vi "sub vi test.vi"() -> ()   [LabVIEW 2019]
uses:
  <userlib>/defectsWrapper/defectsWrapper.lvlib
panel:
  out "Image":T1(plugin-control)
  in  "margin":dbl[][](array[numeric])=[[650.0, 1550.0]]
  in  "thr":dbl[][](array[numeric])=[[900.0, 900.0, 1000.0, 1100.0, 1800.0, 1800.0, 2000.0, 2200.0]]
  in  "File Path":path
  in  "error in (no error)":errorcluster
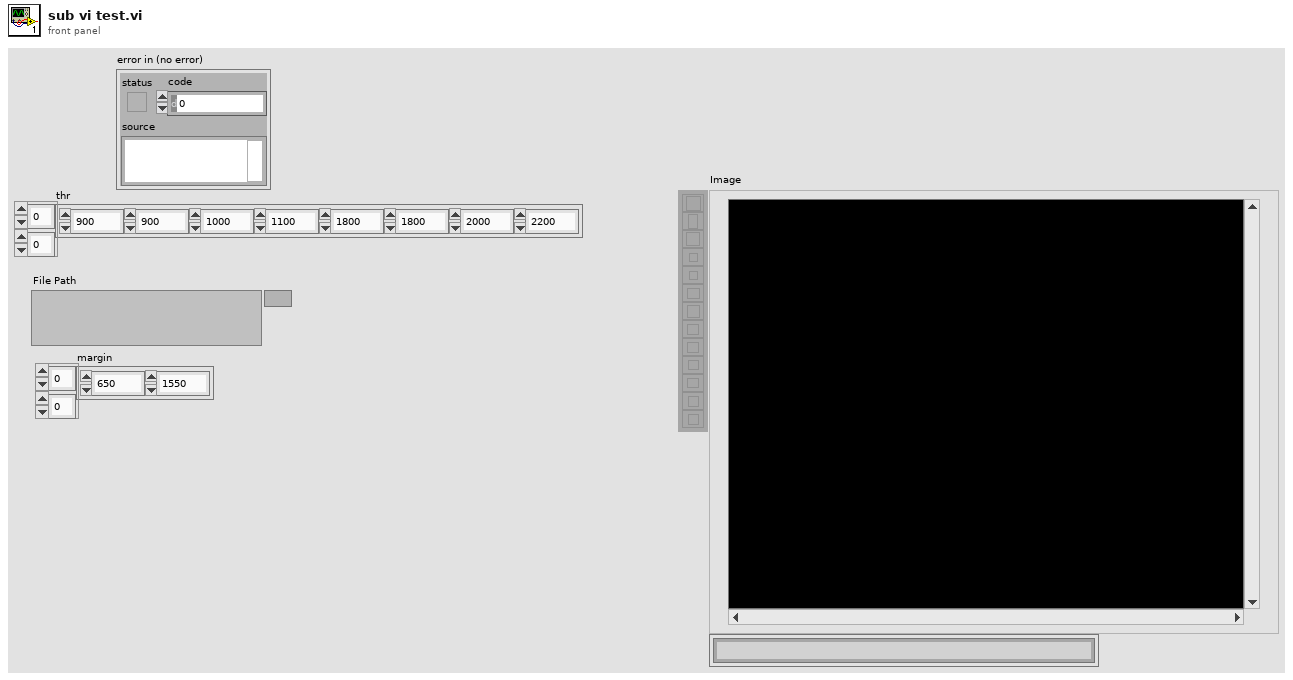
[diagram p1: front panel]
types:
  T1 = typedef "IMAQ Image.ctl" = refnum<image>
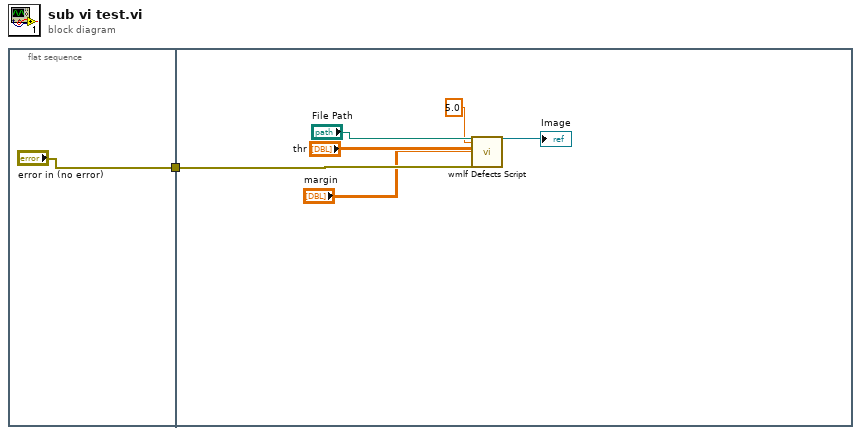
[diagram p0: block diagram]
diagram:
  n1 = flat-sequence {
    tunnel: ["error in (no error)"] -> w1
    tunnel: w1 -> [w8]
    frame #0 {
    }
    frame #1 {
      n2 = call <userlib>:"wmlf Defects Script.vi"("File Path"="File Path", "size"=5.0, "threshoulds"="thr", "margin"="margin", "error in (no error)"=w8) -> ("Image"=→"Image":T1)  [unwired: 16 in, 6 out]
    }
  }
